vi "solar_misc Email Config.vi"(5 "Action (Read)":enum8{"Read", "Write"}(ring), 7 "Section (\"\" = Filename)":string, 8 "error in (no error)":errorcluster, 9 "Key Prefix ('email_')":string="email_", 10 "Config in":T1={"Enabled"=FALSE, "MailServer"="mail.aero.ball.com", "MailServerPort"=25, "EmailTimeout"=5000, "ReturnAddress"="batcsolar@ball.com", "Recipients"=[], "Subject"="SOLAR Email Notification"}, 11 "Email.ini":path) -> (0 "error out":errorcluster, 2 "Config out":T1={"Enabled"=FALSE, "MailServer"="mail.aero.ball.com", "MailServerPort"=25, "EmailTimeout"=5000, "ReturnAddress"="batcsolar@ball.com", "Recipients"=[], "Subject"=""}, 3 "dup Email.ini":path)   [LabVIEW 2018]
doc: "This loads the Email configuration settings."
uses:
  solar_misc_ctl Email Config.ctl
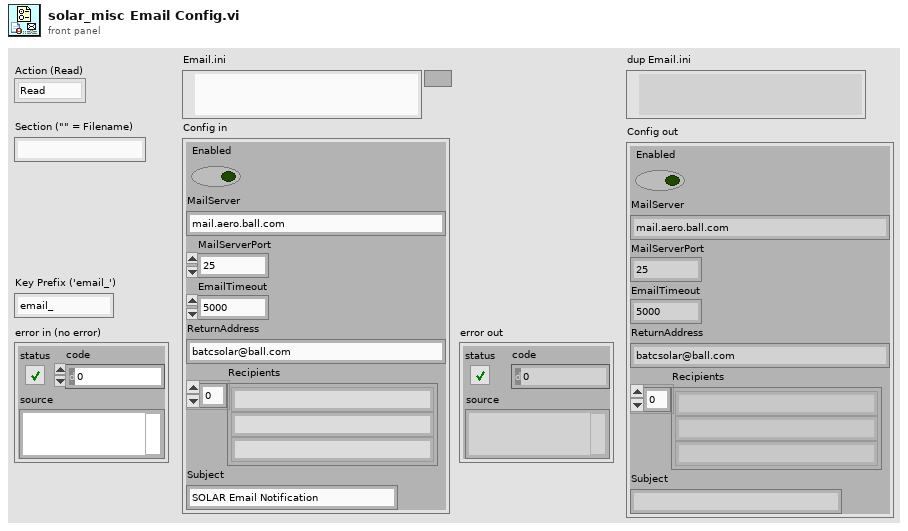
[diagram p1: front panel]
types:
  T1 = typedef "solar_misc_ctl Email Config.ctl" = cluster{"Enabled":bool, "MailServer":string, "MailServerPort":u16, "EmailTimeout":i32, "ReturnAddress":string, "Recipients":string[], "Subject":string}
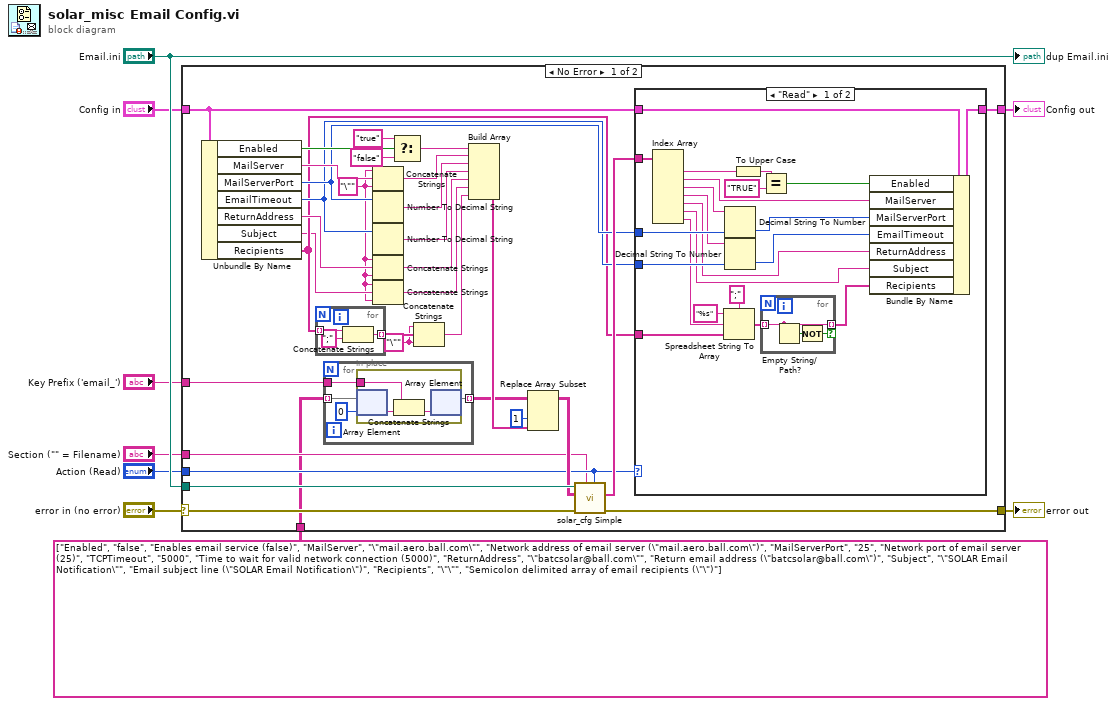
[diagram p0: block diagram]
diagram:
  n1 = case shown="No Error" "error in (no error)" {
    selector: "error in (no error)" -> [w42 w80]
    tunnel: "Email.ini" -> [w41 _]
    tunnel: "Config in" -> [w40 w79]
    tunnel: [w26 w80] -> w6
    tunnel: [w35 w79] -> w5
    tunnel: "Action (Read)" -> [w14 _]
    tunnel: string[][] [["Enabled", "false", "Enables email service (false)"], ["MailServer", "\"mail.aero.ball.com\"", "Network address of email server (\"mail.aero.ball.com\")"], ["MailServerPort", "25", "Network port of email server (25)"], ["TCPTimeout", "5000", "Time to wait for valid network connection (5000)"], ["ReturnAddress", "\"batcsolar@ball.com\"", "Return email address (\"batcsolar@ball.com\")"], ["Subject", "\"SOLAR Email Notification\"", "Email subject line (\"SOLAR Email Notification\")"], ["Recipients", "\"\"", "Semicolon delimited array of email recipients (\"\")"]] ("Key,Value,Comment") -> [w12 _]
    tunnel: "Section (\"\" = Filename)" -> [w13 _]
    tunnel: "Key Prefix ('email_')" -> [w10 _]
    frame No Error {
      w15 = "\"" ("string")
      w18 = "\"" ("string")
      n2 = Unbundle By Name(w40) -> ("Enabled"=w39:bool, "MailServer"=w36:string, "MailServerPort"=w33:u16, "EmailTimeout"=w32:i32, "ReturnAddress"=w31:string, "Subject"=w19:string, "Recipients"=w21:string[])
      n3 = for {
        tunnel: w21 -> [w78] mode=indexing
        tunnel: [w76] -> w20 mode=indexing
        n4 = Concatenate Strings(w78, ";" ("string")) -> (w76:string)
      }
      n5 = for {
        tunnel: w12 -> [w46] mode=indexing
        tunnel: [w45] -> w11 mode=indexing
        tunnel: w10 -> [w43]
        n6 = in-place {
          in-place-border: w43 -> [w47]
          n7 = in-place-array #1(w46, 0) -> (w49:string)
          n8 = Concatenate Strings(w47, w49) -> (w48:string)
          n9 = in-place-array #1(w48) -> (w45:string[])  [unwired: 1 out]
        }
      }
      n10 = Concatenate Strings(w18, w36, w18) -> (w25:string)
      n11 = Number To Decimal String(number=w33) -> (decimal integer string=w24:string)  [unwired: 1 in]
      n12 = Number To Decimal String(number=w32) -> (decimal integer string=w23:string)  [unwired: 1 in]
      n13 = Concatenate Strings(w18, w31, w18) -> (w22:string)
      n14 = Concatenate Strings(w18, w19, w18) -> (w17:string)
      n15 = Select(t="true", s=w39, f="false") -> (s? t:f=w28:string)
      n16 = Concatenate Strings(w15, w20, w15) -> (w16:string)
      n17 = Build Array(w28, w25, w24, w23, w22, w17, w16) -> (w27:string[])
      n18 = Replace Array Subset(array=w11, new element=w27, index (col)=1 ("disabled index (col)")) -> (w29:string[][])  [unwired: 1 in]
      n19 = call "solar_cfg Simple.vi"("Action (Read)"=w14, "Section (\"\" = Filename)"=w13, "error in (no error)"=w42, "Key,Value,Comment"=w29, "Config Path (*.ini)"=w41) -> ("error out"=w26:errorcluster, "Values"=w34:string[])  [unwired: 3 in, 2 out]
      n20 = case shown="\"Read\"" w14 {
        tunnel: w40 -> [w71 w75]
        tunnel: [w70 w75] -> w35
        tunnel: w34 -> [w69 _]
        tunnel: w33 -> [w64 _]
        tunnel: w32 -> [w63 _]
        tunnel: w21 -> [w55 _]
        frame "Read" {
          n21 = Index Array(array=w69) -> (element #1=w59:string, element #2=w58:string, element #3=w57:string, element #4=w56:string, element #5=w54:string, element #6=w53:string, element #7=w52:string)  [unwired: 7 in]
          n22 = Spreadsheet String To Array(delimiter (Tab)=";", format string="%s", spreadsheet string=w52, array type (2D Dbl)=w55) -> (array=w51:string[])
          n23 = Decimal String To Number(string=w57, default (0L)=w64) -> (number=w65:u16)  [unwired: 1 in, 1 out]
          n24 = Decimal String To Number(string=w56, default (0L)=w63) -> (number=w62:i32)  [unwired: 1 in, 1 out]
          n25 = To Upper Case(1:w59) -> (0:w68:string)
          n26 = Equal?(x=w68, y="TRUE") -> (x = y?=w66:bool)
          n27 = for {
            tunnel: w51 -> [w74] mode=indexing
            tunnel: [w74] -> w50 mode=indexing if=w72
            n28 = Empty String/Path?(string/path=w74) -> (empty?=w73:bool)
            n29 = Not(x=w73) -> (.not. x?=w72:bool)
          }
          n30 = Bundle By Name(cluster=w71, "Enabled"=w66, "MailServer"=w58, "MailServerPort"=w65, "EmailTimeout"=w62, "ReturnAddress"=w54, "Subject"=w53, "Recipients"=w50) -> (w70:T1)
        }
        frame "Write" {
        }
      }
    }
    frame Error {
    }
  }
  "error out" <- w6
  "Config out" <- w5
  "dup Email.ini" <- "Email.ini"
